vi "XML.IntoArray.vi"(8 "error in":errorcluster, 10 "XML file path":path) -> (0 "error out":errorcluster, 2 "Config":T1[](array[typedef]))   [LabVIEW 2019, in "Tools.lvlib"]
uses:
  Tools.lvlib
  <vilib>/xml/NI_XML.lvlib
  <vilib>/xml/Load XML File.vi
  Modules/Sequences_Management/SubVIs/ConfigurationWizard/controls/ConfigurationWIzard.Config.ctl
  <vilib>/xml/Close Reference(Node).vi
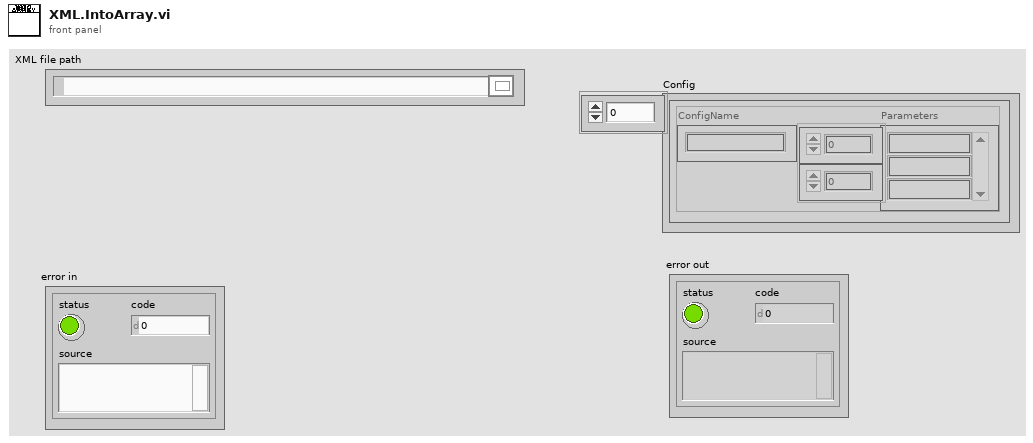
[diagram p1: front panel]
types:
  T1 = typedef "ConfigurationWIzard.Config.ctl" = cluster{"ConfigName":string, "Parameters":string[][]}
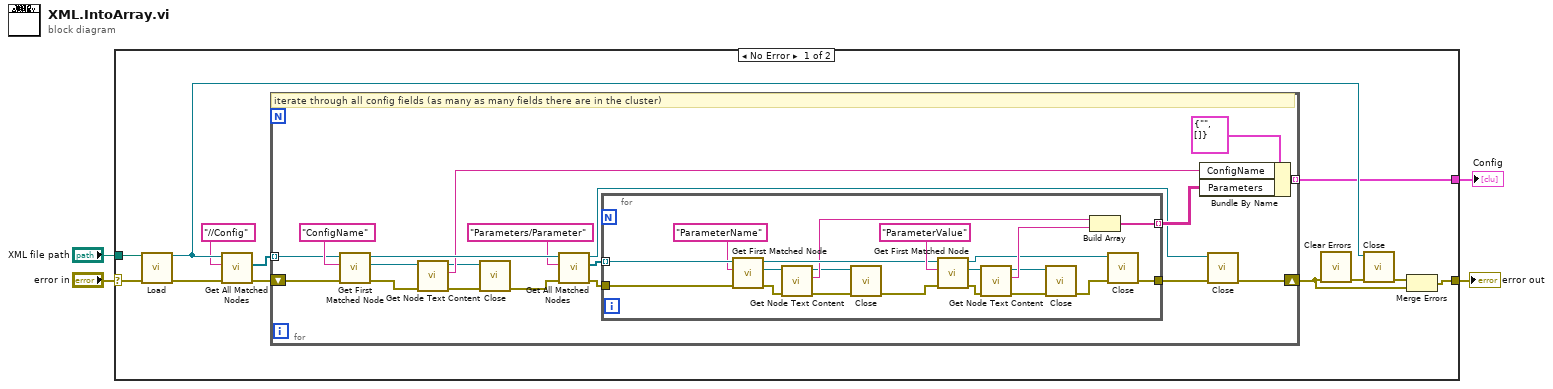
[diagram p0: block diagram]
diagram:
  n1 = case shown="No Error" "error in" {
    selector: "error in" -> [w15 w56]
    tunnel: [w13 w56] -> w4
    tunnel: "XML file path" -> [w16 _]
    tunnel: [w5 _] -> w1
    frame No Error {
      n2 = call-poly <vilib>:"Load.vi"("path to XML document"=w16, "error in (no error)"=w15) -> ("DOM document out"=w14:refnum<k20>, "error out"=w8:errorcluster)  [unwired: 11 in, 1 out]
      n3 = call <vilib>:"Get All Matched Nodes.vi"("error in (no error)"=w8, "XPath expression"="//Config", "node in"=w14) -> ("error out"=w11:errorcluster, "node result array"=w10:refnum<k20>[])  [unwired: 6 in, 1 out]
      n4 = for {
        tunnel: w10 -> [w25] mode=indexing
        shift-right: [w18] -> w7
        shift-left: w11 -> [w35]
        tunnel: [w22] -> w5 mode=indexing
        # "iterate through all config fields (as many as many fields there are in the cluster)"
        n5 = call <vilib>:"Get First Matched Node.vi"("error in (no error)"=w35, "XPath expression"="ConfigName", "node in"=w25) -> ("error out"=w32:errorcluster, "node result"=w33:refnum<k20>, "node out"=w31:refnum<k20>)  [unwired: 6 in]
        n6 = call <vilib>:"Get Node Text Content.vi"("error in (no error)"=w32, "node in"=w33) -> ("error out"=w28:errorcluster, "node text"=w23:string, "node out"=w19:refnum<k20>)  [unwired: 7 in]
        n7 = call-poly <vilib>:"Close.vi"("error in (no error)"=w28, "node"=w19) -> ("error out"=w20:errorcluster)  [unwired: 7 in]
        n8 = call <vilib>:"Get All Matched Nodes.vi"("error in (no error)"=w20, "XPath expression"="Parameters/Parameter", "node in"=w31) -> ("error out"=w27:errorcluster, "node result array"=w29:refnum<k20>[], "node out"=w17:refnum<k20>)  [unwired: 6 in]
        n9 = for {
          tunnel: w29 -> [w55] mode=indexing
          tunnel: w27 -> [w51]
          tunnel: [w37] -> w26
          tunnel: [w42] -> w24 mode=indexing
          n10 = call <vilib>:"Get First Matched Node.vi"("error in (no error)"=w51, "XPath expression"="ParameterName", "node in"=w55) -> ("error out"=w49:errorcluster, "node result"=w50:refnum<k20>, "node out"=w52:refnum<k20>)  [unwired: 6 in]
          n11 = call <vilib>:"Get Node Text Content.vi"("error in (no error)"=w49, "node in"=w50) -> ("error out"=w48:errorcluster, "node text"=w46:string, "node out"=w40:refnum<k20>)  [unwired: 7 in]
          n12 = call-poly <vilib>:"Close.vi"("error in (no error)"=w48, "node"=w40) -> ("error out"=w41:errorcluster)  [unwired: 7 in]
          n13 = call <vilib>:"Get First Matched Node.vi"("error in (no error)"=w41, "XPath expression"="ParameterValue", "node in"=w52) -> ("error out"=w47:errorcluster, "node result"=w45:refnum<k20>, "node out"=w36:refnum<k20>)  [unwired: 6 in]
          n14 = call <vilib>:"Get Node Text Content.vi"("error in (no error)"=w47, "node in"=w45) -> ("error out"=w44:errorcluster, "node text"=w43:string, "node out"=w38:refnum<k20>)  [unwired: 7 in]
          n15 = call-poly <vilib>:"Close.vi"("error in (no error)"=w44, "node"=w38) -> ("error out"=w39:errorcluster)  [unwired: 7 in]
          n16 = Build Array(w46, w43) -> (w42:string[])
          n17 = call-poly <vilib>:"Close.vi"("error in (no error)"=w39, "node"=w36) -> ("error out"=w37:errorcluster)  [unwired: 7 in]
        }
        n18 = Bundle By Name(cluster=T1 {"ConfigName"="", "Parameters"=[]} ("Config"), "ConfigName"=w23, "Parameters"=w24) -> (w22:T1)
        n19 = call-poly <vilib>:"Close.vi"("error in (no error)"=w26, "node"=w17) -> ("error out"=w18:errorcluster)  [unwired: 7 in]
      }
      n20 = call <vilib>:"Clear Errors.vi"("error in (no error)"=w7) -> ("error out"=w6:errorcluster)  [unwired: 5 in, 1 out]
      n21 = call-poly <vilib>:"Close.vi"("error in (no error)"=w6, "node"=w14) -> ("error out"=w12:errorcluster)  [unwired: 7 in]
      n22 = Merge Errors(w12, w7) -> (w13:errorcluster)
    }
    frame Error {
    }
  }
  "error out" <- w4
  "Config" <- w1
